vi "Format Query.vi"(1 "CMD in":string) -> (0 "CMD out":string)   [LabVIEW 2020]
uses:
  MS_Global.vi
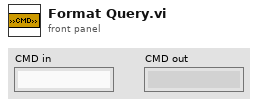
[diagram p1: front panel]
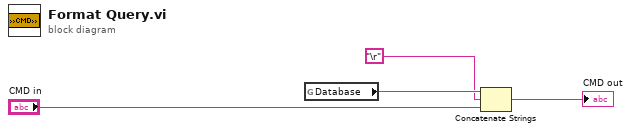
[diagram p0: block diagram]
diagram:
  n1 = global read "MS_Global.vi" "Database"() -> (w4:string)
  n2 = Concatenate Strings(w4, "\r", "CMD in") -> (→"CMD out":string)
